vi "Local2Global Target Values.vi"(6 "Direction":enum16{" +", " - "}(ring)=enum." - ", 11 "Target  Inputs":T1[](array[typedef])) -> (3 "Target  Outputs":T1[](array[typedef]))   [LabVIEW 2009]
uses:
  Target.ctl
  Data Access Objects/Metadata/LBCB Number.ctl
  Apps/App Status Actions.ctl
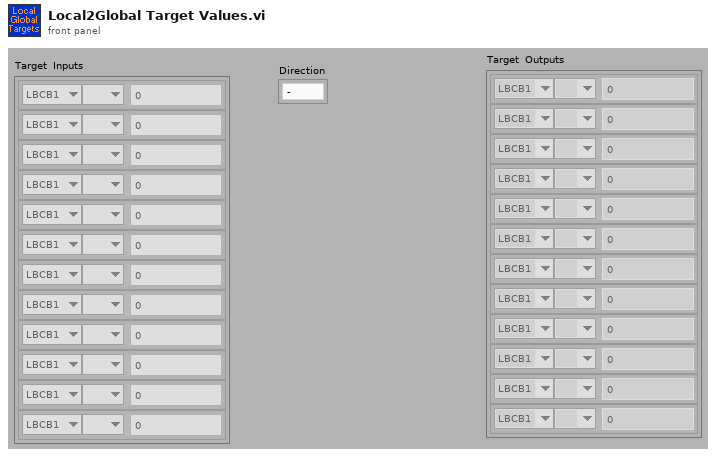
[diagram p1: front panel]
types:
  T1 = typedef "Target.ctl" = cluster{"LBCB Number":T2, "DOF Vectors":enum16{" ", "Dx", "Dy", "Dz", "Rx", "Ry", "Rz", "Fx", "Fy", "Fz", "Mx", "My", "Mz"}, "Amount":dbl}
  T2 = typedef "LBCB Number.ctl" = enum16{"LBCB1", "LBCB2"}
  T3 = typedef "App Status Actions.ctl" = enum16{"Init", "Get Status", "Running", "Control", "Autobalanced", "Data Acquisition", "Set App State", "DAQ Started", "Set LBCB State", "Set All", "Set Cont Logging", "Set Step Logging", "Set MM Logging", "Set Volt Logging", "Set Cart Type", "Set DAQ Link", "Set NTCP Link"}
  T4 = typedef "App Status.ctl" = cluster{"Running":bool, "Controlling L2":bool, "Autobalance L2":bool, "Data Acquisition":bool, " App State":T5, "DAQ Started":bool, "LBCB 1 State":T6, "LBCB 2 State":T6, "Controlling L1":bool, "Autobalance L1":bool, "Cartesian Type":bool, "Continuous Logging":bool, "Step Logging":bool, "Voltage Logging":bool, "Mixed Mode Logging":bool, "DAQ Link":bool, "NTCP Link ":bool}
  T5 = typedef "AppStates.ctl" = enum16{"Starting OM", "Initializing Displays", "Setting up Archiving", "Setting Up DAQ Channels", "Start DAQ", "DAQ Starting", "Controlling LBCBs", "Stopping OM"}
  T6 = typedef "Lbcb Control Loop States.ctl" = enum16{"Idle", "Start Selected", "Load Last Command", "Start Autobalancing", "Autobalancing", "Control Loop Initialized", "Control Enabled"}
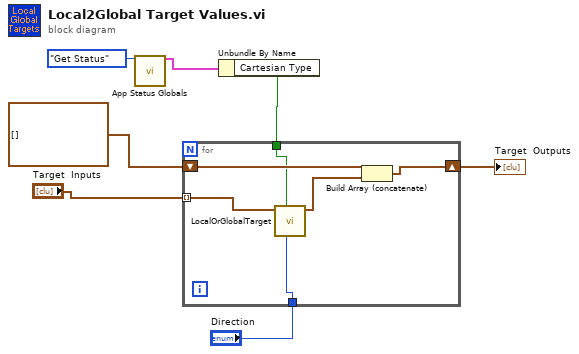
[diagram p0: block diagram]
diagram:
  n1 = call "App Status Globals.vi"("App Status Actions"=App_Status_Actions."Get Status") -> ("App Status Out"=w4:T4)  [unwired: 5 in, 9 out]
  n2 = Unbundle By Name(w4) -> ("Cartesian Type"=w3:bool)
  n3 = for {
    tunnel: "Target  Inputs" -> [w13] mode=indexing
    shift-right: [w10] -> w5
    shift-left: T1[] [] -> [w11]
    tunnel: w3 -> [w9]
    tunnel: "Direction" -> [w8]
    n4 = call "LocalOrGlobalTarget.vi"("Direction"=w8, "Cartesian Type"=w9, "Target"=w13) -> ("Adjusted Target"=w12:T1)  [unwired: 8 in]
    n5 = Build Array (concatenate)(w11, w12) -> (w10:T1[])
  }
  "Target  Outputs" <- w5
